vi "Find_calibration_file.vi"(1 "Inst type":T1=enum."Pressure Transducer", 2 "Ch No":string, 3 "Use Latest Calib":bool, 4 "filename":path) -> (0 "filename out":path)   [LabVIEW 2013]
uses:
  Controls/Inst_type.ctl
  Controls/App_Global.ctl
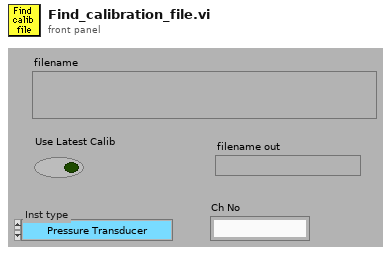
[diagram p1: front panel]
types:
  T1 = typedef "Inst_type.ctl" = enum16{"Propeller anemometer", "Raw voltage", "Pressure Transducer", "Pitot-static tube", "Preston tube", "Hot wire", "Cross wire 1", "Cross wire 2", "Generic Linear", "Generic Polynomial", "Generic BackPoly", "Fast FID", "Thermocouple", "Cold wire", "Pulsed Wire", "LDA Vel", "LDA Tran time", "LDA Arr time"}
  T2 = typedef "App_Global.ctl" = enum16{"Read Global", "Write to Global", "Initialise Array"}
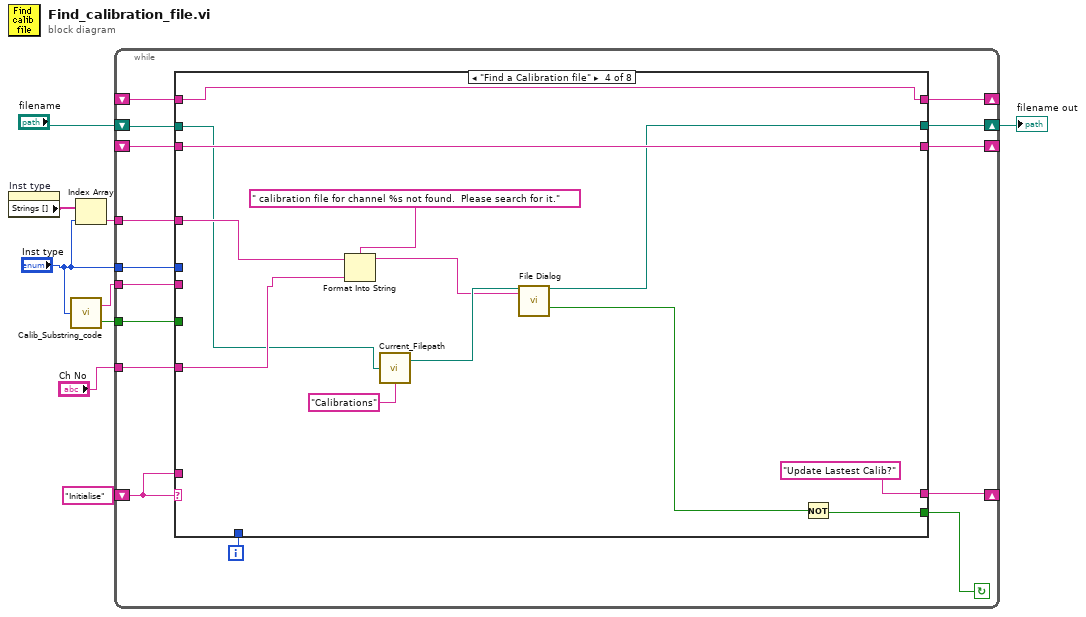
[diagram p0: block diagram]
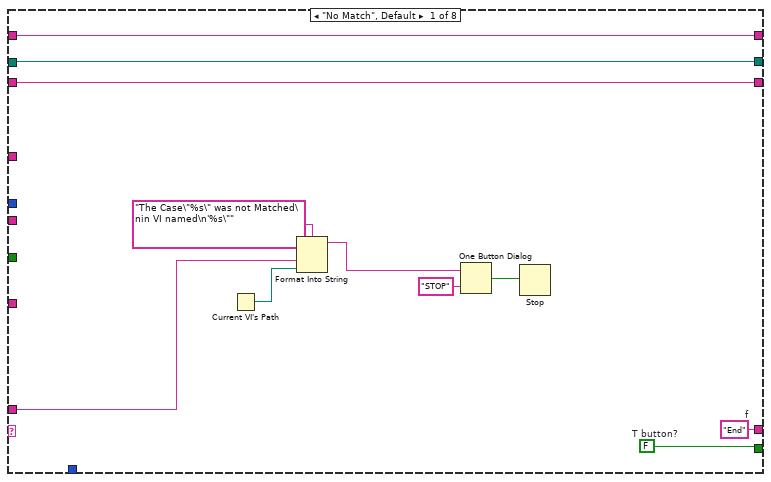
[diagram p2: hidden frame]
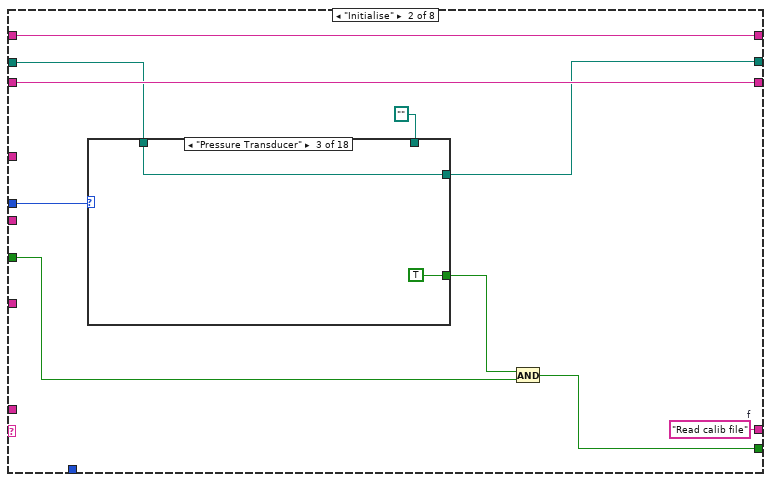
[diagram p3: hidden frame]
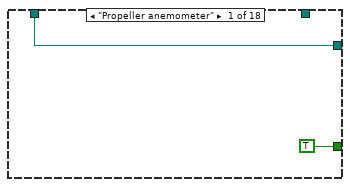
[diagram p4: hidden frame]
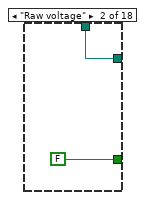
[diagram p5: hidden frame]
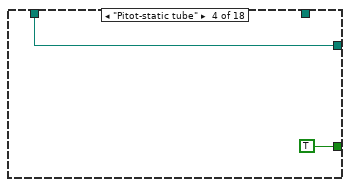
[diagram p6: hidden frame]
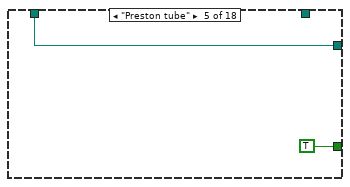
[diagram p7: hidden frame]
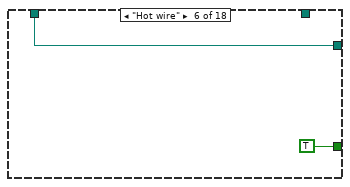
[diagram p8: hidden frame]
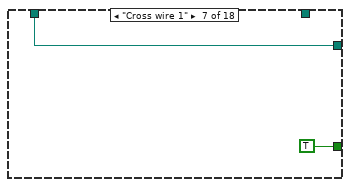
[diagram p9: hidden frame]
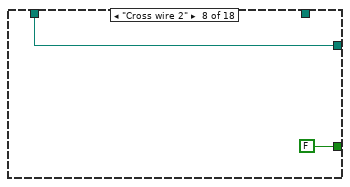
[diagram p10: hidden frame]
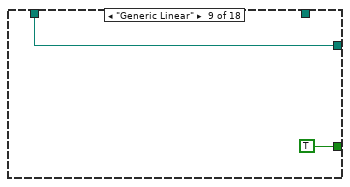
[diagram p11: hidden frame]
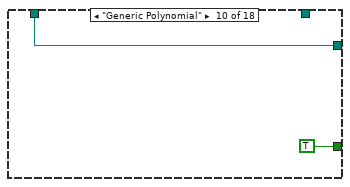
[diagram p12: hidden frame]
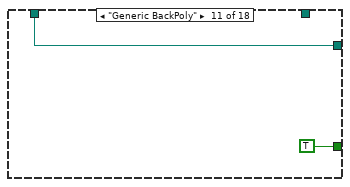
[diagram p13: hidden frame]
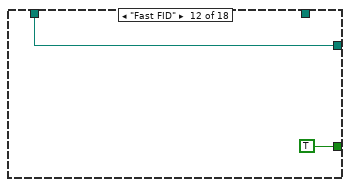
[diagram p14: hidden frame]
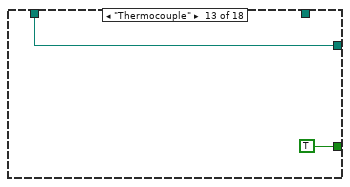
[diagram p15: hidden frame]
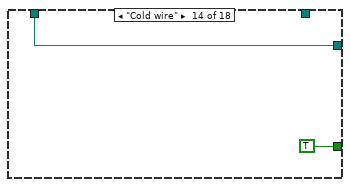
[diagram p16: hidden frame]
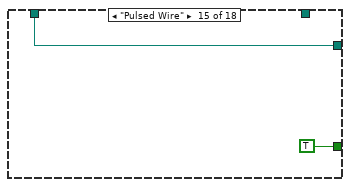
[diagram p17: hidden frame]
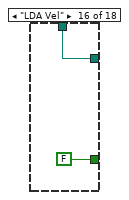
[diagram p18: hidden frame]
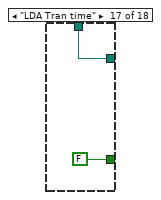
[diagram p19: hidden frame]
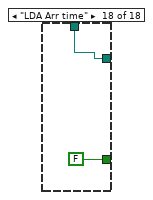
[diagram p20: hidden frame]
diagram:
  n1 = property on="Inst type" class="Enum (strict)"() -> ("Strings []"=w6:string[])  [unwired: 2 in, 2 out]
  n2 = call "Calib_Substring_code.vi"("Inst type"="Inst type") -> ("Substring Type"=w3:string, "Read file"=w2:bool)
  n3 = Index Array(array=w6, index="Inst type") -> (element=w5:string)
  n4 = while {
    shift-left: "filename" -> [w24]
    shift-right: [w23] -> w8
    shift-left: "Initialise" -> [w17]
    shift-right: [w22] -> _
    shift-right: [w19] -> _
    shift-left: _ -> [w18]
    tunnel: "Inst type" -> [w16]
    tunnel: w5 -> [w15]
    shift-right: [w13] -> _
    shift-left: _ -> [w14]
    tunnel: w3 -> [w12]
    tunnel: w2 -> [w11]
    tunnel: "Ch No" -> [w10]
    i -> [w20]
    stop <- w21 continue-if-true
    n5 = case shown="\"Find a Calibration file\"" w17 {
      tunnel: w24 -> [w34 w40 w89 w94 w104 w126 w159 w188]
      tunnel: [w34 w41 w89 w91 w104 w126 w159 w188] -> w23
      tunnel: [w33 w42 w85 "Update Lastest Calib?" w109 w138 "Find a Calibration file" "Read calib file" ("f")] -> w22
      tunnel: [w32 w36 TRUE w100 w112 w139 w174 w186] -> w21
      tunnel: w20 -> [_ _ _ _ _ _ _ _]
      tunnel: [w35 w45 w84 w102 w107 w136 w161 w190] -> w19
      tunnel: w18 -> [w35 w45 _ w102 w107 w136 w161 w190]
      tunnel: w17 -> [w26 _ _ _ _ _ _ _]
      tunnel: w16 -> [_ w43 _ _ _ w137 _ _]
      tunnel: w15 -> [_ _ _ w98 w110 _ _ _]
      tunnel: w14 -> [w25 w44 w82 w99 _ w135 w162 w189]
      tunnel: [w25 w44 w82 w99 w108 w135 w162 w189] -> w13
      tunnel: w12 -> [_ _ _ _ w106 _ _ _]
      tunnel: w11 -> [_ w37 _ _ _ _ _ _]
      tunnel: w10 -> [_ _ _ w96 _ _ _ w185]
      frame "No Match", Default {
        w32 = FALSE  # T button?
        w33 = "End"  # f
        n6 = Current VI's Path() -> (path=w27:path)
        n7 = Format Into String(format string="The Case\"%s\" was not Matched\nin VI named\n'%s\"" ("Format String"), w26, w27) -> (resulting string=w30:string)  [unwired: 2 in, 1 out]
        n8 = One Button Dialog(message=w30, button name ("OK")="STOP") -> (true=w28:bool)
        n9 = Stop(stop? (T)=w28) -> ()
      }
      frame "Initialise" {
        w42 = "Read calib file"  # f
        n10 = case shown="\"Pressure Transducer\"" w43 {
          tunnel: [TRUE FALSE TRUE TRUE TRUE TRUE TRUE FALSE TRUE TRUE TRUE TRUE TRUE TRUE TRUE FALSE FALSE FALSE] -> w38
          tunnel: [w46 w48 w50 w52 w54 w56 w58 w60 w62 w64 w66 w68 w70 w72 w74 w76 w78 w80] -> w41
          tunnel: w40 -> [w46 _ w50 w52 w54 w56 w58 w60 w62 w64 w66 w68 w70 w72 w74 _ _ _]
          tunnel: path "" -> [_ w48 _ _ _ _ _ _ _ _ _ _ _ _ _ w76 w78 w80]
          frame "Propeller anemometer" {
          }
          frame "Raw voltage" {
          }
          frame "Pressure Transducer" {
          }
          frame "Pitot-static tube" {
          }
          frame "Preston tube" {
          }
          frame "Hot wire" {
          }
          frame "Cross wire 1" {
          }
          frame "Cross wire 2" {
          }
          frame "Generic Linear" {
          }
          frame "Generic Polynomial" {
          }
          frame "Generic BackPoly" {
          }
          frame "Fast FID" {
          }
          frame "Thermocouple" {
          }
          frame "Cold wire" {
          }
          frame "Pulsed Wire" {
          }
          frame "LDA Vel" {
          }
          frame "LDA Tran time" {
          }
          frame "LDA Arr time" {
          }
        }
        n11 = And(x=w38, y=w37) -> (x .and. y?=w36:bool)
      }
      frame "Read calib file" {
        w83 = "Check for calib substring"  # f
        n12 = call "Read_File_Simple.vi"("Filename"=w89) -> ("Error?"=w87:bool, "string"=w84:string)  [unwired: 2 in, 6 out]
        n13 = Select(t="Find a Calibration file", s=w87, f=w83) -> (s? t:f=w85:string)
      }
      frame "Find a Calibration file" {
        n14 = Format Into String(format string=" calibration file for channel %s not found.  Please search for it.", initial string=w98, w96) -> (resulting string=w90:string)  [unwired: 1 in, 1 out]
        n15 = call "Current_Filepath.vi"("Filename in"=w94, "Data Type"="Calibrations") -> ("Directory"=w93:path)  [unwired: 1 out]
        n16 = call "File Dialog"("start path"=w93, "prompt"=w90) -> ("selected path"=w91:path, "cancelled"=w92:bool)  [unwired: 10 in, 2 out]
        n17 = Not(x=w92) -> (.not. x?=w100:bool)
      }
      frame "Check for calib substring" {
        w114 = FALSE  # Show Dialog?
        n18 = Concatenate Strings(w106, "calib label") -> (w111:string)
        n19 = Format Into String(format string="Calibration File   %s", w104) -> (resulting string=w103:string)  [unwired: 2 in, 1 out]
        n20 = call "Get_string_subset.vi"("String Name"=w103, "Show Dialog?"=w114, "String to split"=w107, "File Label"=w111) -> ("Status"=w113:enum16{"Char in string", "Char not in string"}, "Output string"=w108:string)
        n21 = case shown="\"Char in string\"" w113 {
          tunnel: [TRUE w123] -> w112
          tunnel: w104 -> [_ w119]
          tunnel: w110 -> [_ w122]
          tunnel: ["Was there sufficient calibration points?" "Find a Calibration file"] -> w109
          frame "Char in string" {
          }
          frame "Char not in string" {
            w120 = "The calibration file\n\"%s\"\nis not the appropriate file for a %s"  # format string
            w124 = "Find another file"  # T button name ("OK")
            n22 = Strip Path(path=w119) -> (name=w118:string)  [unwired: 1 out]
            n23 = Format Into String(format string=w120, w118, w122) -> (resulting string=w125:string)  [unwired: 2 in, 1 out]
            n24 = Two Button Dialog(message=w125, 2:w124) -> (T button?=w123:bool)  [unwired: 1 out]
          }
        }
      }
      frame "Was there sufficient calibration points?" {
        n25 = Format Into String(format string="Calibration File   %s", w126) -> (resulting string=w127:string)  [unwired: 2 in, 1 out]
        n26 = call "2D_array_from_string.vi"("String Name"=w127, "Input string"=w135, "Array title"="Calib points label") -> ("2D data array"=w134:dbl[][])  [unwired: 1 in]
        n27 = for {
          tunnel: w134 -> [w145] mode=indexing
          tunnel: [w141] -> w130 mode=indexing
          n28 = Index Array(array=w145, index=5) -> (element=w143:dbl)
          n29 = Not A Number/Path/Refnum?(number/path/refnum=w143) -> (NaN/Path/Refnum?=w142:bool)
          n30 = Not(x=w142) -> (.not. x?=w141:bool)
        }
        n31 = Boolean To (0,1)(Boolean=w130) -> (0, 1=w133:i16[])
        n32 = Add Array Elements(numeric array=w133) -> (sum=w131:i16)
        n33 = Greater?(x=w131, y=i16 1) -> (0:w129:bool)
        n34 = case shown="True" w129 {
          tunnel: [w150 w154] -> w139
          tunnel: w126 -> [w147 _]
          tunnel: ["Find a Calibration file" "Are XW psi 1 and 2 valid"] -> w138
          tunnel: w137 -> [_ w155]
          frame False {
            w148 = "The calibration file\n\"%s\"\nhas less than two calibration points."  # format string
            w151 = "Find another file"  # T button name ("OK")
            n35 = Strip Path(path=w147) -> (name=w146:string)  [unwired: 1 out]
            n36 = Format Into String(format string=w148, w146) -> (resulting string=w152:string)  [unwired: 2 in, 1 out]
            n37 = Two Button Dialog(message=w152, 2:w151) -> (T button?=w150:bool)  [unwired: 1 out]
          }
          frame True {
            n38 = case shown="\"Propeller anemometer\", Default" w155 {
              tunnel: [FALSE TRUE] -> w154
              frame "Propeller anemometer", Default {
              }
              frame "Cross wire 1" {
              }
            }
          }
        }
      }
      frame "Are XW psi 1 and 2 valid" {
        w167 = FALSE  # Show Dialog?
        n39 = Build Array("C0", "C1", "C2") -> (w169:string[])
        n40 = Format Into String(format string="Calibration File   %s", w159) -> (resulting string=w158:string)  [unwired: 2 in, 1 out]
        n41 = call "Get_string_subset.vi"("String Name"=w158, "Show Dialog?"=w167, "String to split"=w161, "File Label"="Auxiliary constants") -> ("Output string"=w168:string)  [unwired: 1 out]
        n42 = for {
          tunnel: w169 -> [w177] mode=indexing
          tunnel: [w176] -> w166 mode=indexing
          tunnel: w168 -> [w175]
          n43 = call "Get_value_from_string.vi"("Input string"=w175, "Variable name"=w177) -> ("Value"=w176:dbl)  [unwired: 1 in, 1 out]
        }
        n44 = Not A Number/Path/Refnum?(number/path/refnum=w166) -> (NaN/Path/Refnum?=w165:bool[])
        n45 = Or Array Elements(Boolean array=w165) -> (logical OR=w164:bool)
        n46 = case shown="False" w164 {
          tunnel: [FALSE w182] -> w174
          tunnel: w159 -> [_ w180]
          frame False {
          }
          frame True {
            n47 = Strip Path(path=w180) -> (name=w179:string)  [unwired: 1 out]
            n48 = Format Into String(format string="The XW calibration file\n\"%s\"\ndoes not have valid angle calibration coefficients.", w179) -> (resulting string=w184:string)  [unwired: 2 in, 1 out]
            n49 = Two Button Dialog(message=w184, 2:"Find another file" ("T button name (\"OK\")")) -> (T button?=w182:bool)  [unwired: 1 out]
          }
        }
      }
      frame "Update Lastest Calib?" {
        w186 = TRUE  # T button?
        n50 = case shown="True" "Use Latest Calib" {
          tunnel: w188 -> [_ w195]
          tunnel: w185 -> [_ w192]
          frame False {
          }
          frame True {
            n51 = Build Array(w195) -> (w193:path[])
            n52 = Build Array(w192) -> (w194:string[])
            n53 = call "Current_Calib_Filenames.vi"("Mode"=App_Global."Write to Global", "Channel Numbers"=w194, "Calib Filename"=w193) -> ()  [unwired: 2 in, 2 out]
          }
        }
      }
    }
  }
  "filename out" <- w8
